vi "sin_grad.vi"(1 "angle out":dbl) -> (0 "Numeric":dbl)   [LabVIEW 2011]
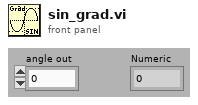
[diagram p1: front panel]
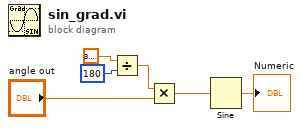
[diagram p0: block diagram]
diagram:
  n1 = Divide(x=3.141592653589793, y=180) -> (x/y=w1:dbl)
  n2 = Multiply(x=w1, y="angle out") -> (x*y=w4:dbl)
  n3 = Sine(x=w4) -> (sin(x)=→"Numeric":dbl)
